vi "UI Initialize.vi"(8 "error in (no error)":errorcluster, 11 "Apply Language Wizard in":refnum<class "Apply Language Wizard.lvclass">) -> (0 "error out":errorcluster, 3 "Apply Language Wizard out":refnum<class "Apply Language Wizard.lvclass">)   [LabVIEW 2013, in "SET Project Editor.lvlib" / "Apply Language Wizard.lvclass"]
uses:
  Apply Language Wizard.lvclass
  UI Wizard/UI Wizard.lvclass/UI Wizard.ctl
  UI Wizard/UI Wizard.lvclass
  Apply Language Wizard.lvclass/Apply Language Wizard.ctl
  SET Project Data/Project Data Class/Project Data.lvclass
  SET Project Data/Project Data Class/Project Data.lvclass/Project Data.ctl
  SET Project Data/Resource Data Class/Resource Data.lvclass/Resource Data.ctl
  SET Project Data/VI Class/VI Data.lvclass
  SET Project Data/Menu Class/Menu Data.lvclass/Menu Data.ctl
  SET Project Data/Menu Class/Read Menu Path (Relative).vi
  SET Project Data/Project Data Class/Read Menu Table.vi
  SET Project Data/Resource Data Class/Read Languages.vi
  UI Wizard/Read Project Data ref.vi
  SET Project Data/Menu Class/Menu Data.lvclass
  SET Project Data/Resource Data Class/Resource Data.lvclass
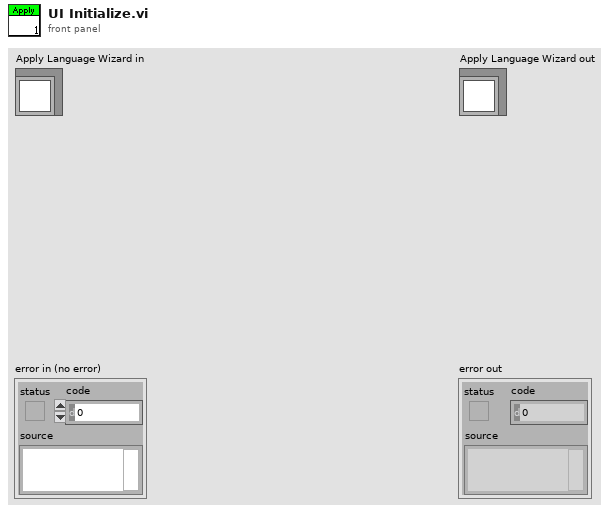
[diagram p1: front panel]
types:
  T1 = enum32{"Invalid", "Default", "Floating", "Floating/Auto-Hide", "Modal"}
  T2 = typedef "SET Project Data.lvlib/ProjFile_Language Data.ctl" = cluster{"Tag":string, "Name":string, "Code Page":u16}
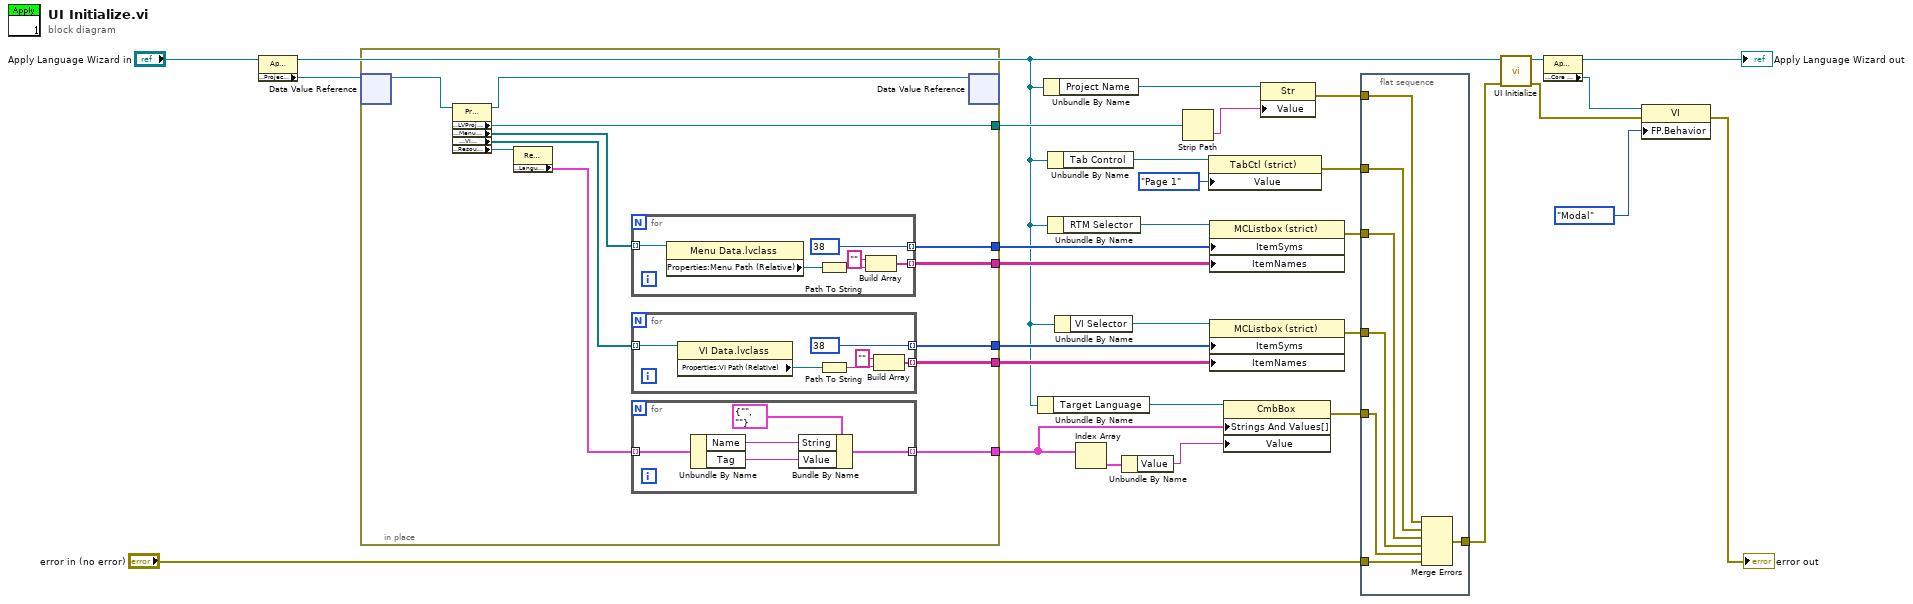
[diagram p0: block diagram]
diagram:
  n1 = property class="Apply Language Wizard.lvclass"(reference="Apply Language Wizard in") -> (reference out=w18:refnum<class "Apply Language Wizard.lvclass">, "Properties:Project Data ref"=w30:refnum<data-value>)  [unwired: 1 in, 1 out]
  n2 = in-place {
    in-place-border: [w40] -> w29
    in-place-border: [w36] -> w23
    in-place-border: [w35] -> w22
    in-place-border: [w34] -> w20
    in-place-border: [w33] -> w19
    in-place-border: [w32] -> w3
    n3 = in-place-dvr #1(w30) -> (w43:refnum<class "Project Data.lvclass">)  [unwired: 1 out]
    n4 = property class="Project Data.lvclass"(reference=w43) -> (reference out=w41:refnum<class "Project Data.lvclass">, "Properties:LVProject File Path"=w40:path, "Properties:Menu Table"=w39:refnum<class "Menu Data.lvclass">[], "Properties:VI Table"=w38:refnum<class "VI Data.lvclass">[], "Properties:Resource Data ref"=w42:refnum<data-value>)  [unwired: 1 in, 1 out]
    n5 = property class="Resource Data.lvclass"(reference=w42) -> ("Properties:Languages []"=w37:T2[])  [unwired: 1 in, 2 out]
    n6 = for {
      tunnel: w39 -> [w60] mode=indexing
      tunnel: [w56] -> w35 mode=indexing
      tunnel: [38] -> w36 mode=indexing
      n7 = property class="Menu Data.lvclass"(reference=w60) -> ("Properties:Menu Path (Relative)"=w59:path)  [unwired: 1 in, 2 out]
      n8 = Path To String(path=w59) -> (string=w58:string)
      n9 = Build Array("" ("element"), w58) -> (w56:string[])
    }
    n10 = for {
      tunnel: w38 -> [w54] mode=indexing
      tunnel: [38] -> w34 mode=indexing
      tunnel: [w49] -> w33 mode=indexing
      n11 = property class="VI Data.lvclass"(reference=w54) -> ("Properties:VI Path (Relative)"=w53:path)  [unwired: 1 in, 2 out]
      n12 = Path To String(path=w53) -> (string=w51:string)
      n13 = Build Array("" ("element"), w51) -> (w49:string[])
    }
    n14 = for {
      tunnel: w37 -> [w48] mode=indexing
      tunnel: [w44] -> w32 mode=indexing
      n15 = Unbundle By Name(w48) -> ("Name"=w46:string, "Tag"=w45:string)
      n16 = Bundle By Name(cluster=cluster{"String":string, "Value":string} {"String"="", "Value"=""}, "String"=w46, "Value"=w45) -> (w44:cluster{"String":string, "Value":string})
    }
    n17 = in-place-dvr #1(w41) -> ()  [unwired: 2 out]
  }
  n18 = Unbundle By Name(w18) -> ("Target Language"=w17:refnum<vi>)
  n19 = Unbundle By Name(w18) -> ("Project Name"=w28:refnum<vi>)
  n20 = Unbundle By Name(w18) -> ("Tab Control"=w25:refnum<vi>)
  n21 = Unbundle By Name(w18) -> ("RTM Selector"=w24:refnum<vi>)
  n22 = Unbundle By Name(w18) -> ("VI Selector"=w21:refnum<vi>)
  n23 = Index Array(array=w3) -> (element=w2:cluster{"String":string, "Value":string})  [unwired: 1 in]
  n24 = Unbundle By Name(w2) -> ("Value"=w1:string)
  n25 = Strip Path(path=w29) -> (name=w27:string)  [unwired: 1 out]
  n26 = property class="TabCtl (strict)"(reference=w25, "Value"=enum32{"Page 1", "Page 2"}."Page 1") -> (error out=w15:errorcluster)  [unwired: 1 in, 1 out]
  n27 = property class="MCListbox (strict)"(reference=w24, "ItemSyms"=w23, "ItemNames"=w22) -> (error out=w14:errorcluster)  [unwired: 1 in, 1 out]
  n28 = property class="MCListbox (strict)"(reference=w21, "ItemSyms"=w20, "ItemNames"=w19) -> (error out=w13:errorcluster)  [unwired: 1 in, 1 out]
  n29 = property class="CmbBox"(reference=w17, "Strings And Values[]"=w3, "Value"=w1) -> (error out=w12:errorcluster)  [unwired: 1 in, 1 out]
  n30 = property class="Str"(reference=w28, "Value"=w27) -> (error out=w16:errorcluster)  [unwired: 1 in, 1 out]
  n31 = flat-sequence {
    tunnel: w16 -> [w62]
    tunnel: w15 -> [w63]
    tunnel: w14 -> [w64]
    tunnel: w13 -> [w65]
    tunnel: w12 -> [w66]
    tunnel: "error in (no error)" -> [w67]
    tunnel: [w61] -> w10
    frame #0 {
      n32 = Merge Errors(w62, w63, w64, w65, w66, w67) -> (w61:errorcluster)
    }
  }
  n33 = call-parent "UI Initialize.vi"("error in (no error)"=w10, "UI Wizard in"=w18) -> ("error out"=w5:errorcluster, "UI Wizard out"=w6:refnum<class "Apply Language Wizard.lvclass">)  [unwired: 8 in]
  n34 = property class="Apply Language Wizard.lvclass"(reference=w6) -> (reference out=→"Apply Language Wizard out":refnum<class "Apply Language Wizard.lvclass">, "Properties:Core VI Refnum"=w8:refnum<vi>)  [unwired: 1 in, 1 out]
  n35 = property class="VI"(reference=w8, error in=w5, "FP.Behavior"=T1."Modal" ("Front Panel Window:Behavior")) -> (error out=→"error out":errorcluster)  [unwired: 1 out]
